vi "CloseTCPIP.vi"(2 "error in (no error)":errorcluster, 3 "connection ID":refnum<k5>) -> (0 "error out":errorcluster)   [LabVIEW 2014]
doc: "Closes a TCPIP connection"
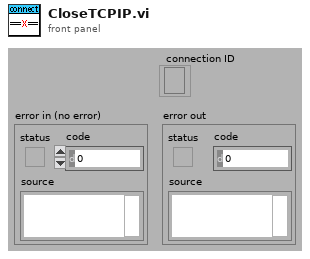
[diagram p1: front panel]
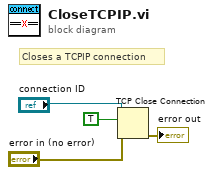
[diagram p0: block diagram]
diagram:
  # "Closes a TCPIP connection"
  n1 = TCP Close Connection(connection ID="connection ID", abort (F)=TRUE, error in (no error)="error in (no error)") -> (error out=→"error out":errorcluster)  [unwired: 1 out]
